vi "IR_Laser_Control.vi"(0 "Action":T1(ring), 5 "Energy (0 - 100)":i16 min=0 max=100, 7 "Rep. Rate Divider":i16, 9 "Command String":string) -> (15 "error_Code":i32)   [LabVIEW 2015]
uses:
  OPOTEK.dll
panel:
  # "LASER CONTROL"
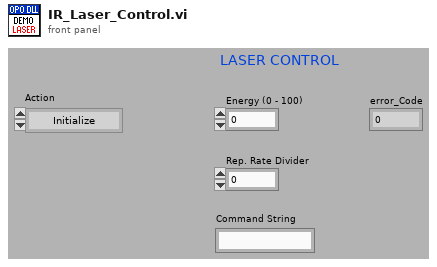
[diagram p1: front panel]
types:
  T1 = enum16{"Initialize", "Lamp ON", "Lamp OFF", "Q-switch ON", "Q-switch OFF", "Adjust Energy", "Change Rep. Rate", "Send String"}
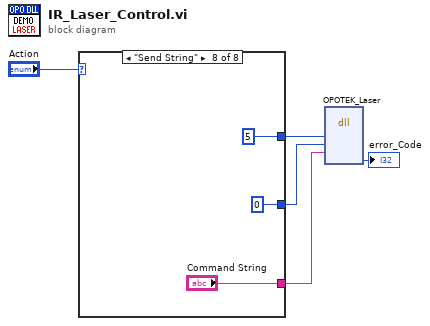
[diagram p0: block diagram]
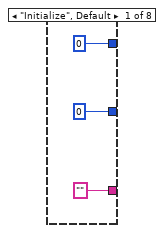
[diagram p2: hidden frame]
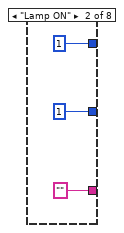
[diagram p3: hidden frame]
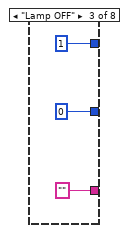
[diagram p4: hidden frame]
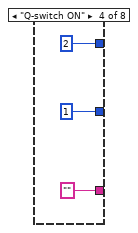
[diagram p5: hidden frame]
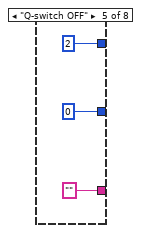
[diagram p6: hidden frame]
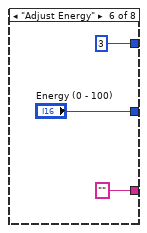
[diagram p7: hidden frame]
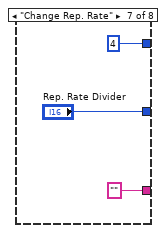
[diagram p8: hidden frame]
diagram:
  n1 = case shown="\"Send String\"" "Action" {
    tunnel: [i8 0 ("action") i8 1 ("action") i8 1 ("action") i8 2 ("action") i8 2 ("action") i8 3 ("action") i8 4 ("action") i8 5 ("action")] -> w3
    tunnel: [i16 0 ("parameter") i16 1 ("parameter") i16 0 ("parameter") i16 1 ("parameter") i16 0 ("parameter") "Energy (0 - 100)" "Rep. Rate Divider" i16 0 ("Rep. Rate Divider")] -> w2
    tunnel: ["" ("stringToSend") "" ("stringToSend") "" ("stringToSend") "" ("stringToSend") "" ("stringToSend") "" ("stringToSend") "" ("stringToSend") "Command String"] -> w1
    frame "Initialize", Default {
    }
    frame "Lamp ON" {
    }
    frame "Lamp OFF" {
    }
    frame "Q-switch ON" {
    }
    frame "Q-switch OFF" {
    }
    frame "Adjust Energy" {
    }
    frame "Change Rep. Rate" {
    }
    frame "Send String" {
    }
  }
  n2 = dll-call lib="Z:/Software/Labview/FD_VIs/IR Opolette Controller/OPOTEK.dll" fn="OPOTEK_Laser"("action"=w3, "parameter"=w2, "stringToSend"=w1) -> ("error_Code"=→"error_Code":i32)  [unwired: 8 in, 2 out]
